vi "RT Main.vi"() -> ()   [LabVIEW 2016]
doc: "The top-level VI for the LabVIEW RIO Eval Kit.\n\nThis VI runs through multiple stages. Each stage demonstrates different features of the RIO Eval Kit. The program uses a State Machine Producer/Consumer architecture. The top loop reads and writes information to and from the FPGA. That information is sent to the bottom through a queue. The information being transfered includes both the data and the type of message being sent. The bottom loop then handles displaying the appropriate information on the LCD."
uses:
  <vilib>/rvi/interface/nirviCloseFPGA/nirviCloseFPGA.xnode
  2- Create FPGA Application/controls/SystemStates.ctl
  <vilib>/EmbeddedDisplay/Hitachi HD44780/Host/HD44780 Host.lvlib
  <vilib>/EmbeddedDisplay/Hitachi HD44780/Common/Control/screen size.ctl
  <vilib>/EmbeddedDisplay/Hitachi HD44780/Common/HD44780 Common.lvlib
  <vilib>/EmbeddedDisplay/Hitachi HD44780/Common/Control/font configuration.ctl
  2- Create FPGA Application/controls/SoundOptions.ctl
  2- Create FPGA Application/controls/Queue Data.ctl
  <vilib>/FPGAPlugInAG/Dynamic/niLvFpga_Close_Dynamic.vi
panel:
  out "Signal":dbl[](graph)
  out "Alarm":bool
  in  "Alarm Threshold":dbl=4.0
  out "Amplitude":dbl format="%#_3g"
  # "Start by turning encoder right to kickoff first stage, and \ncontinue turning right to complete all three stages. Stop \nthe program at any time by pressing the right button (PB2)."
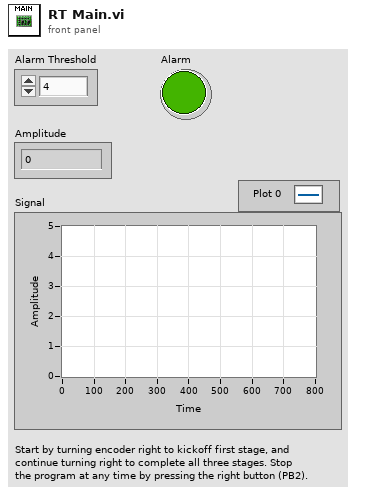
[diagram p1: front panel]
types:
  T1 = typedef "Queue Data.ctl" = cluster{"Current Pos > Threshold?":bool, "Current Pos > Previous?":bool, "Amplitude":dbl, "Stage Number":string}
  T2 = typedef "HD44780 Common.lvlib/font configuration.ctl" = enum8{"5x8 & 2 lines", "5x10 & 1 line", "5x8 & 1 line"}
  T3 = typedef "HD44780 Common.lvlib/screen size.ctl" = enum8{"8x1", "8x2", "12x4", "16x1", "16x2", "16x4", "20x1", "20x2", "20x4", "24x1", "24x2", "40x2", "40x4"}
  T4 = typedef "SystemStates.ctl" = enum16{"Shutdown", "Stage 1", "Stage 2", "Stage 3", "Alarm State"}
  T5 = typedef "SoundOptions.ctl" = enum16{"Ding", "Boing", "Buzzer", "Horn"}
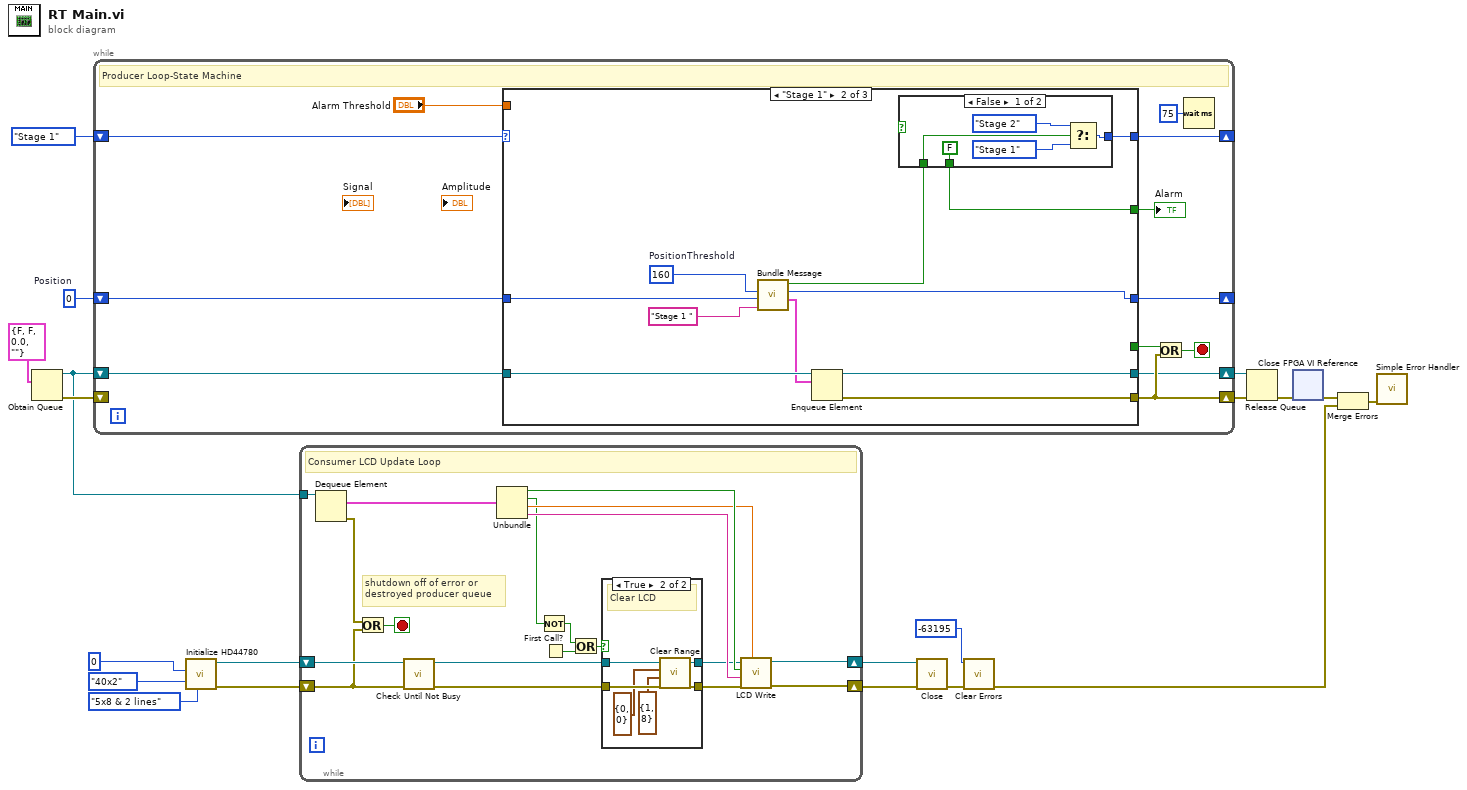
[diagram p0: block diagram]
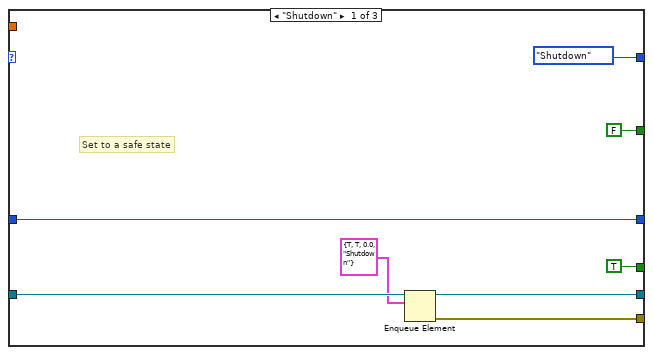
[diagram p3: hidden frame]
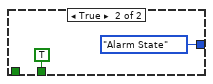
[diagram p4: hidden frame]
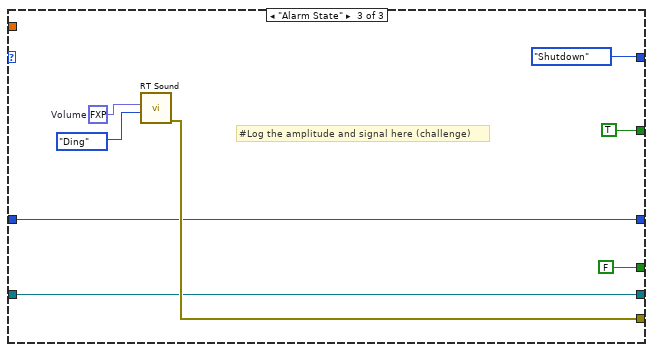
[diagram p5: hidden frame]
diagram:
  w1 = i16 0  # Position
  n1 = Obtain Queue(element data type=T1 {"Current Pos > Threshold?"=FALSE, "Current Pos > Previous?"=FALSE, "Amplitude"=0.0, "Stage Number"=""} ("output to queue")) -> (queue out=w2:refnum<queue>, error out=w4:errorcluster)  [unwired: 4 in, 1 out]
  n2 = while {
    shift-right: [w26] -> w19
    shift-left: w4 -> [_]
    shift-right: [w24] -> w20
    shift-left: w2 -> [w32]
    shift-right: [w28] -> _
    shift-left: SystemStates."Stage 1" ("Enum") -> [w29]
    shift-right: [w21] -> _
    shift-left: w1 -> [w27]
    stop <- w30 stop-if-true
    # "Producer Loop-State Machine"
    n3 = case shown="\"Stage 1\"" w29 {
      tunnel: w32 -> [w37 w51 w62]
      tunnel: [w38 w50 w66] -> w26
      tunnel: [TRUE _ FALSE ("E-Stop")] -> w25
      tunnel: [SystemStates."Shutdown" ("Enum") w49 SystemStates."Shutdown" ("Enum")] -> w28
      tunnel: w27 -> [w34 w43 w59]
      tunnel: [w36 w45 w62] -> w24
      tunnel: [FALSE w44 TRUE] -> w23
      tunnel: "Alarm Threshold" -> [_ _ _]
      tunnel: [w34 w42 w59] -> w21
      frame "Shutdown" {
        # "Set to a safe state"
        n4 = Enqueue Element(queue=w37, element=T1 {"Current Pos > Threshold?"=TRUE, "Current Pos > Previous?"=TRUE, "Amplitude"=0.0, "Stage Number"="Shutdown"} ("output to queue")) -> (queue out=w36:refnum<queue>, error out=w38:errorcluster)  [unwired: 2 in, 1 out]
      }
      frame "Stage 1" {
        w46 = i16 160  # PositionThreshold
        n5 = call "Bundle Message.vi"("Stage Number"="Stage 1 " ("text"), "Previous Position"=w43, "Position Threshold"=w46) -> ("Output to queue"=w41:T1, "Output Position"=w42:i16, "x >= y?"=w48:bool)  [unwired: 6 in]
        n6 = Enqueue Element(queue=w51, element=w41) -> (queue out=w45:refnum<queue>, error out=w50:errorcluster)  [unwired: 2 in, 1 out]
        n7 = case shown="False" {
          selector: _ -> [_ _]
          tunnel: [w54 SystemStates."Alarm State" ("Enum")] -> w49
          tunnel: w48 -> [w53 _]
          tunnel: [FALSE TRUE] -> w44
          frame False {
            n8 = Select(t=SystemStates."Stage 2" ("Enum"), s=w53, f=SystemStates."Stage 1" ("Enum")) -> (s? t:f=w54:T4)
          }
          frame True {
          }
        }
      }
      frame "Alarm State" {
        w64 = fxp<+/-,32,16> 5.0  # Volume
        # "#Log the amplitude and signal here (challenge)"
        n9 = call "RT Sound.vi"("Sound Options"=SoundOptions."Ding" ("Enum"), "Volume"=w64) -> ("error out"=w66:errorcluster)  [unwired: 8 in, 1 out]
      }
    }
    "Alarm" <- w23
    n10 = Or(x=w25, y=w26) -> (x .or. y?=w30:bool)
    n11 = Wait (ms)(milliseconds to wait=u32 75) -> ()  [unwired: 1 out]
  }
  n12 = call <vilib>:"Initialize HD44780.vi"("font configuration (5x8 & 2 lines)"=font_configuration."5x8 & 2 lines", "screen size"=screen_size."40x2", "device index"=i8 0) -> ("error out"=w12:errorcluster, "LCD out"=w13:refnum<class "Character LCD.lvclass">)  [unwired: 7 in]
  n13 = while {
    shift-right: [w68] -> w11
    shift-left: w13 -> [w85]
    shift-right: [w67] -> w10
    shift-left: w12 -> [w84]
    tunnel: w2 -> [w83]
    stop <- w76 stop-if-true
    # "shutdown off of error or \ndestroyed producer queue"
    # "Consumer LCD Update Loop"
    n14 = Dequeue Element(queue=w83) -> (element=w79:T1, error out=w80:errorcluster)  [unwired: 2 in, 2 out]
    n15 = Or(x=w80, y=w84) -> (x .or. y?=w76:bool)
    n16 = call "Check Until Not Busy.vi"("error in"=w84, "LCD in"=w85) -> ("error out"=w77:errorcluster, "LCD out"=w78:refnum<class "Character LCD.lvclass">)  [unwired: 8 in]
    n17 = Unbundle(w79) -> ("Current Pos > Threshold?"=w82:bool, "Current Pos > Previous?"=w72:bool, "Amplitude"=w75:dbl, "Stage Number"=w81:string)
    n18 = Not(x=w72) -> (.not. x?=w69:bool)
    n19 = First Call?() -> (First Call?: T/F=w70:bool)
    n20 = Or(x=w69, y=w70) -> (x .or. y?=w71:bool)
    n21 = case shown="True" w71 {
      tunnel: w78 -> [w87 w93]
      tunnel: w77 -> [w86 w92]
      tunnel: [w86 w91] -> w73
      tunnel: [w87 w90] -> w74
      frame False {
      }
      frame True {
        # "Clear LCD"
        n22 = call <vilib>:"Clear Range.vi"("error in (no error)"=w92, "end position (end of line)"=cluster{"row":i8, "column":i8} {"row"=1, "column"=8} ("start position"), "start position"=cluster{"row":i8, "column":i8} {"row"=0, "column"=0}, "LCD in"=w93) -> ("error out"=w91:errorcluster, "LCD out"=w90:refnum<class "Character LCD.lvclass">)  [unwired: 6 in]
      }
    }
    n23 = call "LCD Write.vi"("Amplitude"=w75, "error in (no error)"=w73, "Stage Number"=w81, "Current Pos > Threshold?"=w82, "Character LCD in"=w74) -> ("error out"=w67:errorcluster, "LCD out"=w68:refnum<class "Character LCD.lvclass">)  [unwired: 4 in]
  }
  n24 = call <vilib>:"Close.vi"("error in (no error)"=w10, "LCD in"=w11) -> ("error out"=w6:errorcluster)  [unwired: 9 in]
  n25 = call <vilib>:"Clear Errors.vi"("error in (no error)"=w6, "specific error code to clear (0: all)"=-63195) -> ("error out"=w5:errorcluster)  [unwired: 4 in, 1 out]
  n26 = Release Queue(queue=w20, error in (no error)=w19) -> (error out=w18:errorcluster)  [unwired: 1 in, 2 out]
  n27 = xnode "Close FPGA VI Reference"("error in"=w18) -> ("error out"=w17:errorcluster)  [unwired: 1 in]
  n28 = Merge Errors(w17, w5) -> (w9:errorcluster)
  n29 = call <vilib>:"Simple Error Handler.vi"("error in (no error)"=w9) -> ()  [unwired: 4 in, 5 out]
